vi "Request Update.vi"(8 "error in (no error)":errorcluster, 11 "ArrayManager in":refnum<class "ArrayManager.lvclass">) -> (0 "error out":errorcluster, 3 "ArrayManager out":refnum<class "ArrayManager.lvclass">)   [LabVIEW 2020, in "OOPanel.lvlib" / "ArrayManager.lvclass"]
uses:
  ArrayManager.lvclass
  ArrayManager.lvclass/ArrayManager.ctl
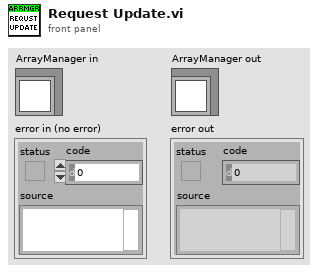
[diagram p1: front panel]
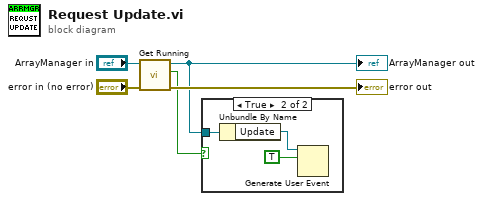
[diagram p0: block diagram]
diagram:
  n1 = call "Get Running.vi"("error in (no error)"="error in (no error)", "ArrayManager in"="ArrayManager in") -> ("error out"=→"error out":errorcluster, "Running"=w2:bool, "ArrayManager out"=w1:refnum<class "ArrayManager.lvclass">)  [unwired: 7 in]
  "ArrayManager out" <- w1
  n2 = case shown="True" w2 {
    tunnel: w1 -> [_ w8]
    frame False {
    }
    frame True {
      n3 = Unbundle By Name(w8) -> ("Update"=w7:refnum<user-event>)
      n4 = Generate User Event(user event=w7, event data cluster=TRUE ("event data")) -> ()  [unwired: 2 in, 2 out]
    }
  }
